vi "read_log_stream.vi"(8 "error in (no error)":errorcluster, 11 "system.logging in":refnum<class "system.logging.lvclass">) -> (0 "error out":errorcluster, 1 "abort?":bool, 2 "log_entry":T1 {"datetime" format="%<%x %.3X>T"}, 3 "system.logging out":refnum<class "system.logging.lvclass">)   [LabVIEW 2021, in "system.logging.lvclass"]
uses:
  system.logging.lvclass
  log_entry.ctl
  severity.ctl
  system.logging.lvclass/system.logging.ctl
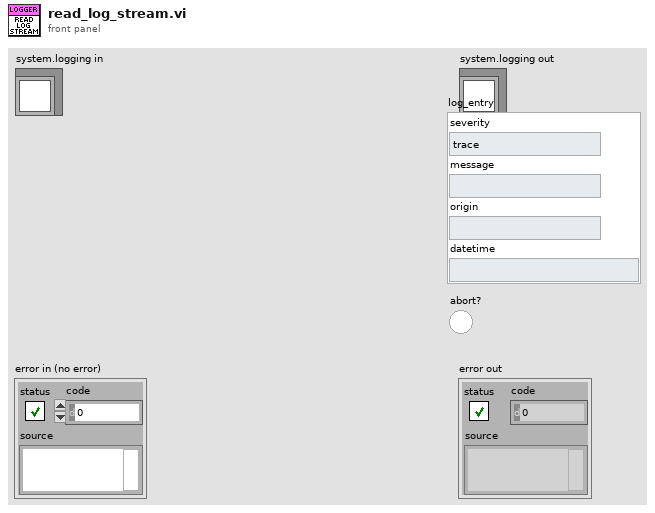
[diagram p1: front panel]
types:
  T1 = typedef "system.logging.lvclass/log_entry.ctl" = cluster{"severity":T2, "message":string, "origin":string, "datetime":timestamp}
  T2 = typedef "system.logging.lvclass/severity.ctl" = enum8{"trace", "debug", "info", "warning", "error"}
  T3 = typedef "system.logging.lvclass/log_stream.ctl" = cluster{"command":T4, "log_entry":T1}
  T4 = typedef "system.logging.lvclass/service_commands.ctl" = enum16{"close", "log"}
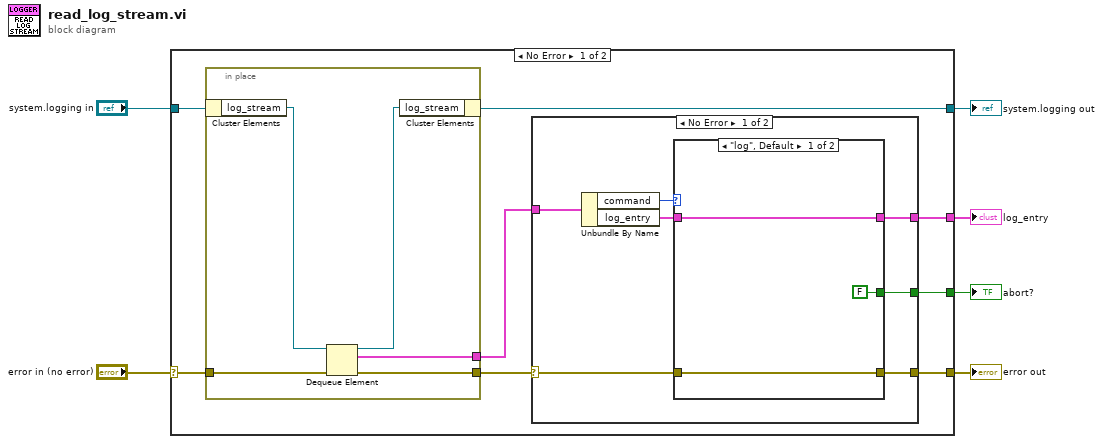
[diagram p0: block diagram]
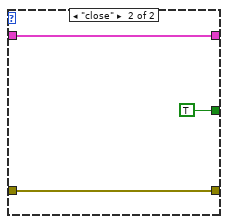
[diagram p2: hidden frame]
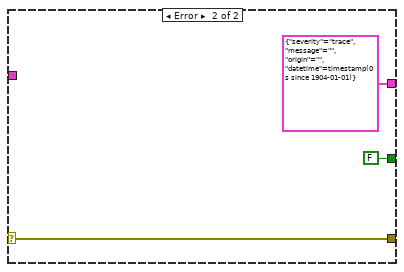
[diagram p3: hidden frame]
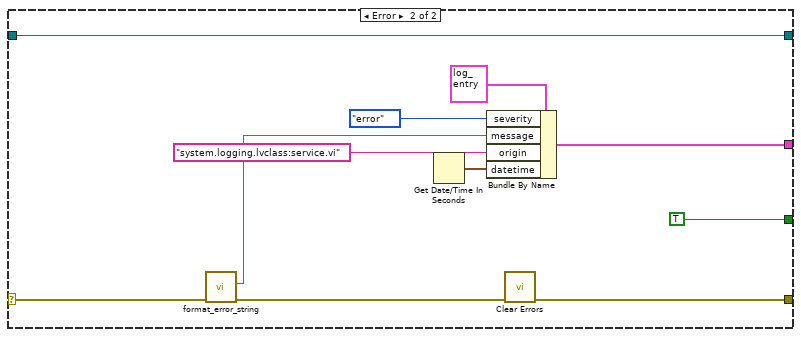
[diagram p4: hidden frame]
diagram:
  n1 = case shown="No Error" "error in (no error)" {
    selector: "error in (no error)" -> [w9 w44]
    tunnel: [w12 w42] -> w5
    tunnel: [w8 w46] -> w3
    tunnel: "system.logging in" -> [w10 w46]
    tunnel: [w11 w37] -> w2
    tunnel: [w13 TRUE ("timed out?")] -> w1
    frame No Error {
      n2 = in-place {
        in-place-border: [w35] -> w14
        in-place-border: [w34] -> w7
        in-place-border: w9 -> [w31]
        n3 = in-place-cluster #1(w10) -> ("log_stream"=w33:refnum<queue>)
        n4 = Dequeue Element(queue=w33, error in (no error)=w31) -> (queue out=w32:refnum<queue>, element=w35:T3, error out=w34:errorcluster)  [unwired: 1 in, 1 out]
        n5 = in-place-cluster #1("log_stream"=w32) -> (w8:refnum<class "system.logging.lvclass">)
      }
      n6 = case shown="No Error" w7 {
        selector: w7 -> [w15 w29]
        tunnel: w14 -> [w21 _]
        tunnel: [w19 FALSE] -> w13
        tunnel: [w18 w29] -> w12
        tunnel: [w17 T1 {"severity"=enum."trace", "message"="", "origin"="", "datetime"=timestamp(0 s since 1904-01-01)} ("log_entry")] -> w11
        frame No Error {
          n7 = Unbundle By Name(w21) -> ("command"=w20:T4, "log_entry"=w16:T1)
          n8 = case shown="\"log\", Default" w20 {
            tunnel: [FALSE TRUE] -> w19
            tunnel: w15 -> [w22 w26]
            tunnel: [w22 w26] -> w18
            tunnel: [w24 w25] -> w17
            tunnel: w16 -> [w24 w25]
            frame "log", Default {
            }
            frame "close" {
            }
          }
        }
        frame Error {
        }
      }
    }
    frame Error {
      n9 = call "format_error_string.vi"("error in (no error)"=w44) -> ("error out"=w43:errorcluster, "error_string"=w38:string)  [unwired: 9 in]
      n10 = Get Date/Time In Seconds() -> (seconds since 1Jan1904=w40:timestamp)
      n11 = Bundle By Name(cluster=T1 {"severity"=enum."trace", "message"="", "origin"="", "datetime"=timestamp(0 s since 1904-01-01)} ("log_entry"), "severity"=severity."error", "message"=w38, "origin"="system.logging.lvclass:service.vi", "datetime"=w40) -> (w37:T1)
      n12 = call <vilib>:"Clear Errors.vi"("error in (no error)"=w43) -> ("error out"=w42:errorcluster)  [unwired: 5 in, 1 out]
    }
  }
  "error out" <- w5
  "system.logging out" <- w3
  "abort?" <- w1
  "log_entry" <- w2
